vi "Get From Type Map.vi"(8 "error in (no error)":errorcluster, 10 "Type Name":string, 11 "TwinCAT ADS in":refnum<class "TwinCAT ADS.lvclass">) -> (0 "error out":errorcluster, 2 ".NET AdsDataType":refnum<k24>, 3 "TwinCAT ADS out":refnum<class "TwinCAT ADS.lvclass">)   [LabVIEW 2018, in "TwinCAT ADS.lvclass"]
uses:
  TwinCAT ADS.lvclass
  TwinCAT.Ads
  TwinCAT ADS.lvclass/TwinCAT ADS.ctl
  <vilib>/Utility/error.llb/Trim Whitespace.vi
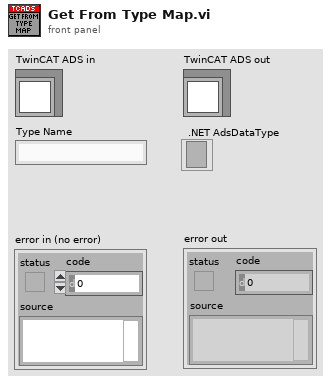
[diagram p1: front panel]
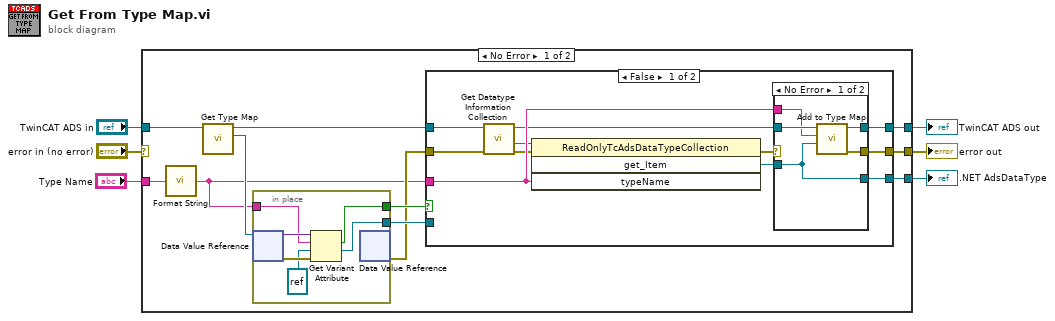
[diagram p0: block diagram]
diagram:
  n1 = case shown="No Error" "error in (no error)" {
    selector: "error in (no error)" -> [_ w45]
    tunnel: "TwinCAT ADS in" -> [w11 w46]
    tunnel: "Type Name" -> [w8 _]
    tunnel: [w15 _] -> w4
    tunnel: [w12 w45] -> w3
    tunnel: [w13 w46] -> w2
    frame No Error {
      n2 = call "Format String.vi"("String"=w8) -> ("Formated String"=w7:string)
      n3 = call "Get Type Map.vi"("TwinCAT ADS in"=w11) -> ("Type Map"=w9:refnum<data-value>, "TwinCAT ADS out"=w10:refnum<class "TwinCAT ADS.lvclass">)  [unwired: 8 in, 1 out]
      n4 = in-place {
        in-place-border: w7 -> [w42]
        in-place-border: [w41] -> w16
        in-place-border: [w40] -> w17
        n5 = in-place-dvr #1(w9) -> (w43:variant, w44:errorcluster)
        n6 = Get Variant Attribute(Variant=w43, name=w42, default value (empty Variant)=refnum<k24> refnum (".NET AdsDataType"), error in=w44) -> (found=w40:bool, value=w41:refnum<k24>)  [unwired: 2 out]
        n7 = in-place-dvr #1() -> (w14:errorcluster)  [unwired: 1 in, 1 out]
      }
      n8 = case shown="False" w17 {
        tunnel: w16 -> [_ w36]
        tunnel: [w25 w36] -> w15
        tunnel: w7 -> [w27 _]
        tunnel: w10 -> [w19 w38]
        tunnel: w14 -> [w18 w37]
        tunnel: [w28 w38] -> w13
        tunnel: [w26 w37] -> w12
        frame False {
          n9 = call "Get Datatype Information Collection.vi"("error in (no error)"=w18, "TwinCAT ADS in"=w19) -> ("error out"=w24:errorcluster, ".NET AdsDatatypeInfoCollection"=w23:refnum<k24>, "TwinCAT ADS out"=w22:refnum<class "TwinCAT ADS.lvclass">)  [unwired: 7 in]
          n10 = invoke class="ReadOnlyTcAdsDataTypeCollection" method="get_Item"(reference=w23, error in=w24, "typeName"=w27) -> (error out=w21:errorcluster, "get_Item"=w20:refnum<k24>)  [unwired: 1 in, 2 out]
          n11 = case shown="No Error" w21 {
            selector: w21 -> [_ w35]
            tunnel: w20 -> [w30 _]
            tunnel: w22 -> [w33 w34]
            tunnel: [w32 w34] -> w28
            tunnel: w27 -> [w29 _]
            tunnel: [w31 w35] -> w26
            tunnel: [w30 _] -> w25
            frame No Error {
              n12 = call "Add to Type Map.vi"(".NET AdsDataType"=w30, "Type Name"=w29, "TwinCAT ADS in"=w33) -> ("error out"=w31:errorcluster, "TwinCAT ADS out"=w32:refnum<class "TwinCAT ADS.lvclass">)  [unwired: 6 in, 1 out]
            }
            frame Error {
            }
          }
        }
        frame True {
        }
      }
    }
    frame Error {
    }
  }
  "error out" <- w3
  "TwinCAT ADS out" <- w2
  ".NET AdsDataType" <- w4
